vi "dispose_.vi"(8 "error in (no error)":errorcluster, 11 "Disposable in":refnum<class "Disposable.lvclass">) -> (0 "error out":errorcluster)   [LabVIEW 2020, in "Lua for LabVIEW.lvlib" / "Disposable.lvclass"]
uses:
  Disposable.lvclass
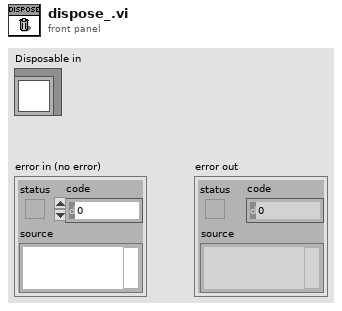
[diagram p1: front panel]
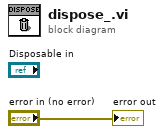
[diagram p0: block diagram]
diagram:
  "error out" <- "error in (no error)"
